vi "BlockDel.vi"() -> ()   [LabVIEW 2019]
uses:
  lib/Snap7.lvlib
panel:
  out "?":string
  in  "BlockType":i32(ring)=67 items=["OB"=56, "DB"=65, "SDB"=66, "FC"=67, "SFC"=68, "FB"=69, "SFB"=70]
  out "Delete Status":string
  in  "Number":i32=1
  in  "Slot":i32=2
  in  "Rack":i32
  in  "Address IP":string="192.168.1.12"
  # "Delete Block"
  # "WARNING !!!\nThis program will delete the selected Block"
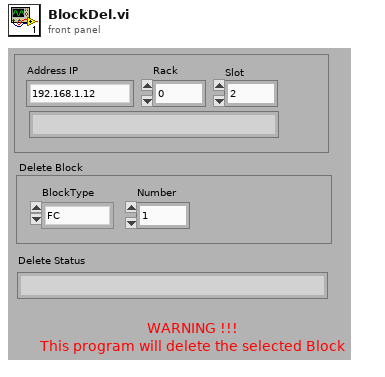
[diagram p1: front panel]
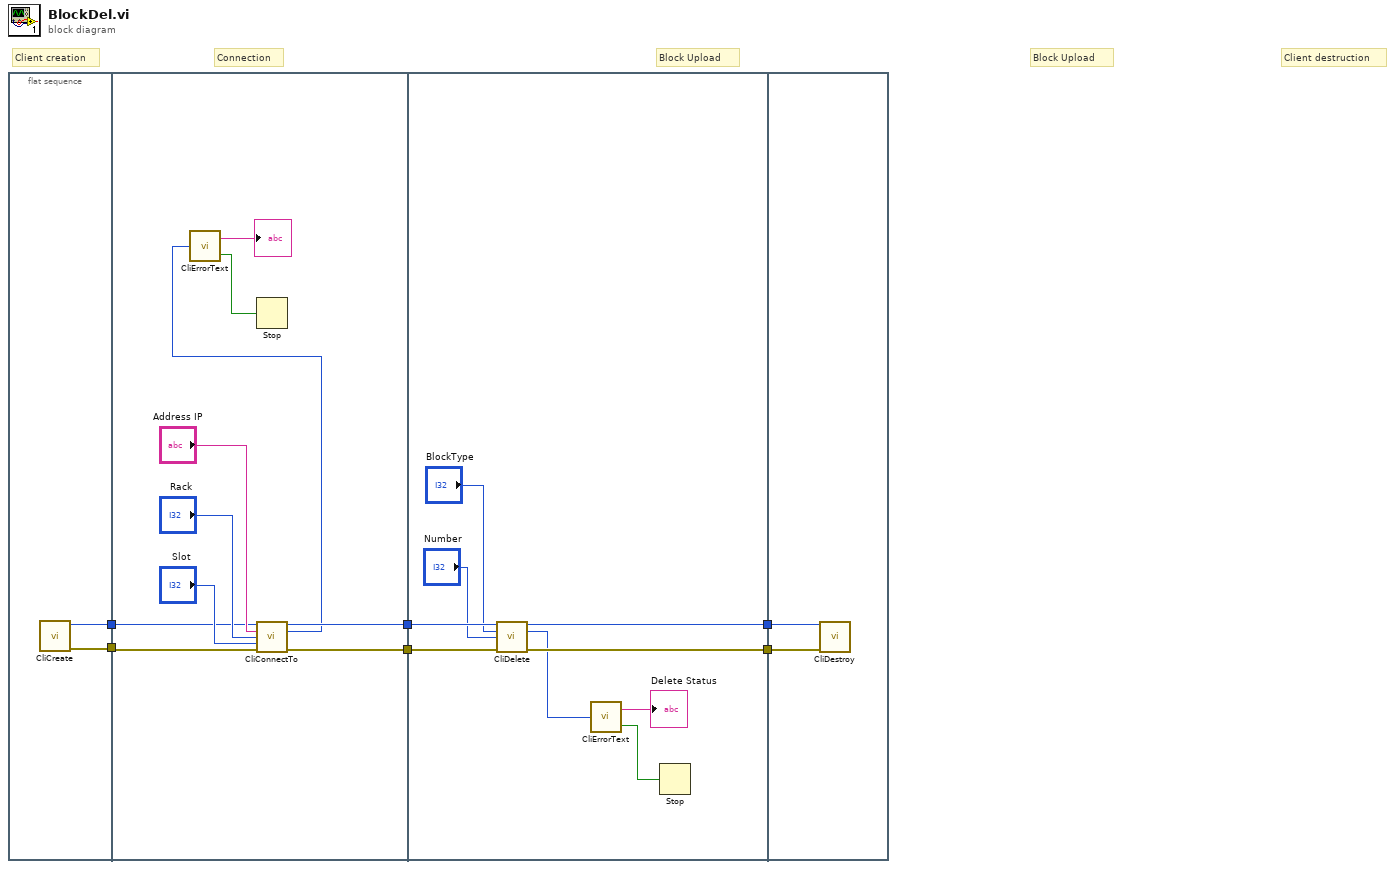
[diagram p0: block diagram]
diagram:
  # "Block Upload"
  # "Client destruction"
  # "Block Upload"
  # "Connection"
  # "Client creation"
  n1 = flat-sequence {
    tunnel: [w8] -> w4
    tunnel: [w7] -> w3
    tunnel: [w18] -> w6
    tunnel: [w12] -> w5
    tunnel: w4 -> [w14]
    tunnel: w3 -> [w13]
    tunnel: w6 -> [w25]
    tunnel: w5 -> [w24]
    tunnel: [w21] -> w2
    tunnel: [w20] -> w1
    tunnel: w2 -> [w29]
    tunnel: w1 -> [w28]
    frame #0 {
      n2 = call "CliCreate.vi"() -> ("ref out"=w8:u64, "error out"=w7:errorcluster)  [unwired: 14 in]
    }
    frame #1 {
      n3 = call "CliConnectTo.vi"("ref in"=w14, "Address"="Address IP", "Rack"="Rack", "Slot"="Slot", "error in (no error)"=w13) -> ("ref out"=w12:u64, "Result"=w9:i32, "error out"=w18:errorcluster)  [unwired: 8 in]
      n4 = call "CliErrorText.vi"("ErrNo"=w9) -> ("Error"=w10:bool, "ErrMessage"=→"?":string)
      n5 = Stop(stop? (T)=w10) -> ()
    }
    frame #2 {
      n6 = call "CliDelete.vi"("ref in"=w24, "BlockType"="BlockType", "Block Number"="Number", "error in (no error)"=w25) -> ("ref out"=w21:u64, "Result"=w19:i32, "error out"=w20:errorcluster)  [unwired: 9 in]
      n7 = call "CliErrorText.vi"("ErrNo"=w19) -> ("Error"=w26:bool, "ErrMessage"=→"Delete Status":string)
      n8 = Stop(stop? (T)=w26) -> ()
    }
    frame #3 {
      n9 = call "CliDestroy.vi"("ref in"=w29, "error in (no error)"=w28) -> ()  [unwired: 13 in, 1 out]
    }
  }
